vi "FORCE_GUIDE.vi"() -> ()   [LabVIEW 2011]
panel:
  in  "Table":string[][](table)=[["20", "9"], ["30", "6"], ["40", "4.5"]]
  in  "BPM":dbl=20.0 caption="Frequency"
  in  "Boolean":bool
  in  "Filename":path=path "C:/Users/Sinha/Desktop/ULLS/140507-RC.csv"
  in  "Target":bool=TRUE
  in  "GUIDE":bool=TRUE
  in  "AI 1":bool=TRUE
  out "?":bool
  in  "AI 0":bool=TRUE
  in  "Target":dbl=1.25 caption="Offset"
  in  "Sample Rate Hz.":dbl=200.0
  out "Waveform Chart":dbl[][](graph)=[[0.1005629623528339, 0.10453920726000487, 1.25, -0.0], [0.10565121703738356, 0.10453920726000487, 1.25, -0.0], [0.09293058032600965, 0.10453920726000487, 1.25, -0.0], [0.1005629623528339, 0.10453920726000487, 1.25, -0.0], [0.1005629623528339, 0.10453920726000487, 1.25, -0.0], [0.1005629623528339, 0.10453920726000487, 1.25, -0.0], [0.10565121703738356, 0.10453920726000487, 1.25, -0.0], [0.09547470766828448, 0.10453920726000487, 1.25, -0.0], [0.09801883501055919, 0.10453920726000487, 1.25, -0.0], [0.1005629623528339, 0.10453920726000487, 1.25, -0.0], [0.10565121703738356, 0.10453920726000487, 1.25, -0.0], [0.09547470766828436, 0.10453920726000487, 1.25, -0.0], [0.09801883501055919, 0.10453920726000487, 1.25, -0.0], [0.09547470766828448, 0.10453920726000487, 1.25, -0.0], [0.10565121703738356, 0.10453920726000487, 1.25, -0.0], [0.10310708969510873, 0.10453920726000487, 1.25, -0.0], [0.10310708969510873, 0.10453920726000487, 1.25, -0.0], [0.1005629623528339, 0.10453920726000487, 1.25, -0.0], [0.10310708969510873, 0.10453920726000487, 1.25, -0.0], [0.10310708969510873, 0.10453920726000487, 1.25, -0.0]]
  in  "save":bool
  in  "stop (F)":bool caption="stop"
  # "USB"
  # "PCI"
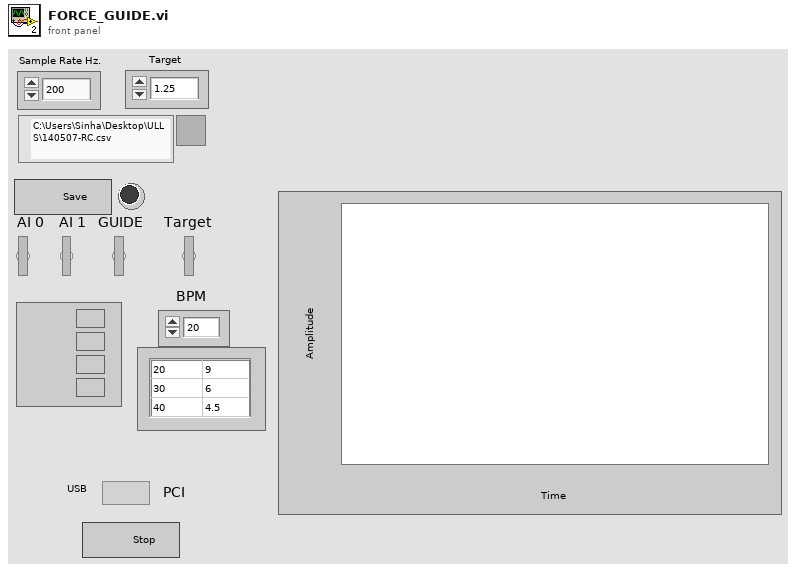
[diagram p1: front panel]
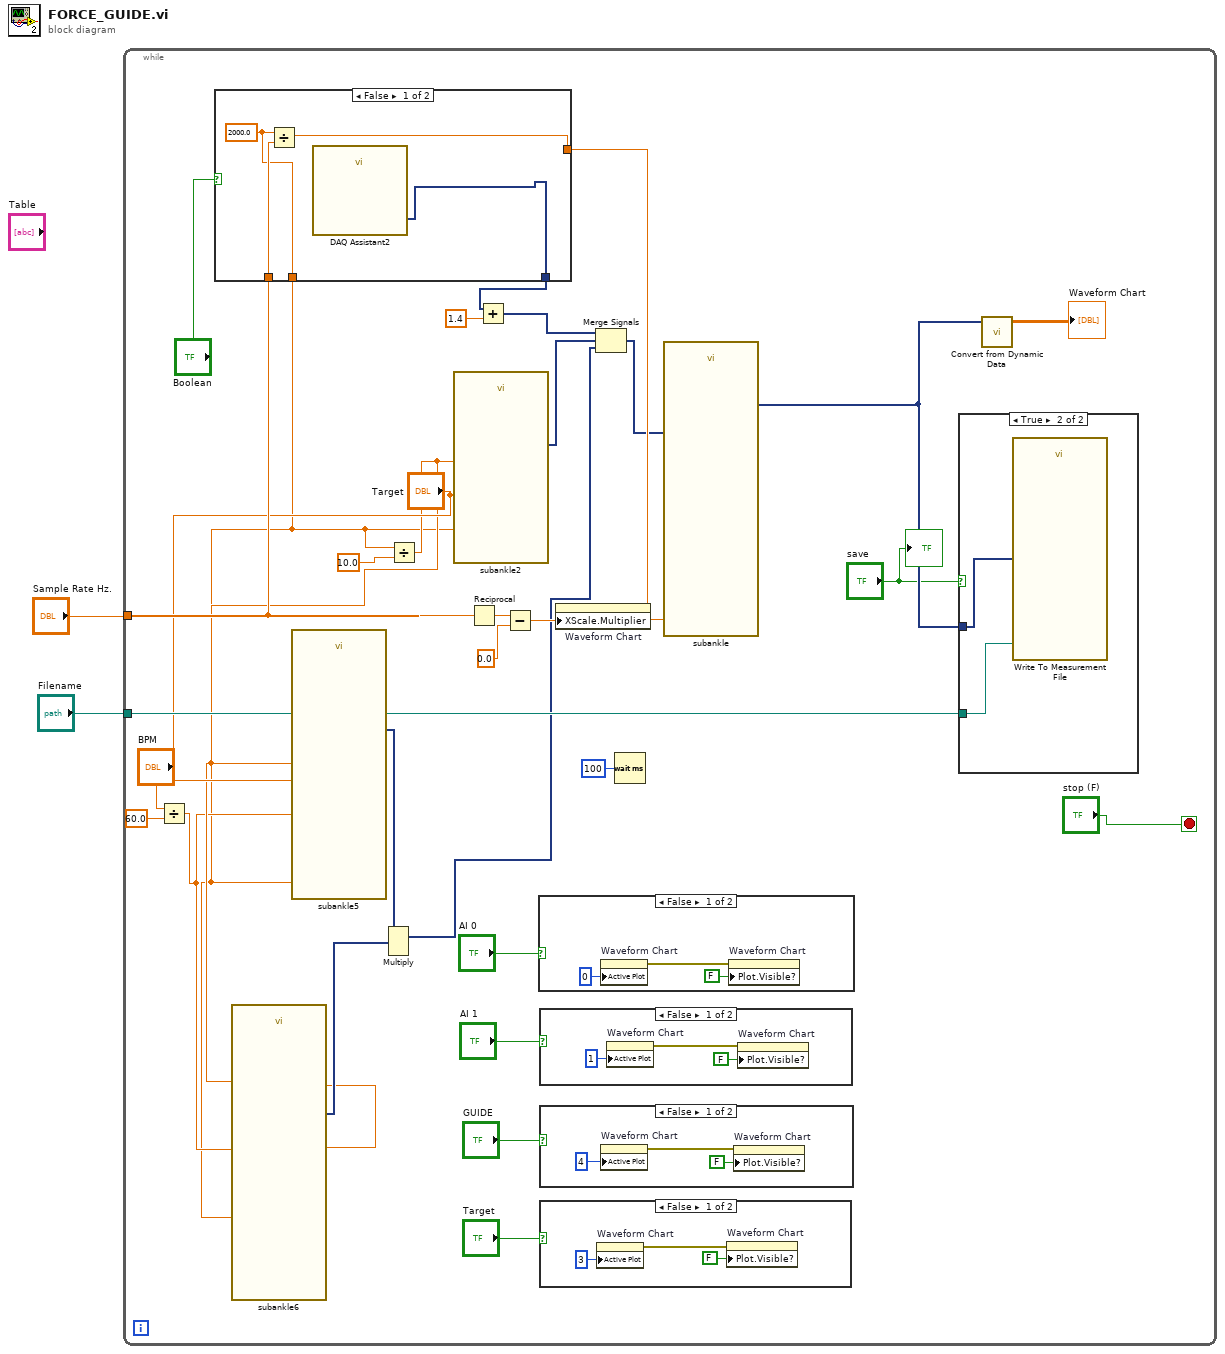
[diagram p0: block diagram]
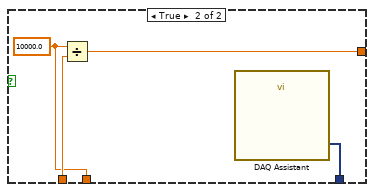
[diagram p2: hidden frame]
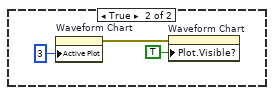
[diagram p3: hidden frame]
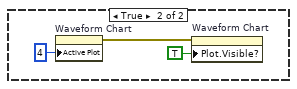
[diagram p4: hidden frame]
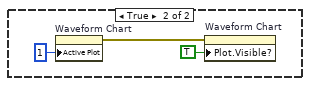
[diagram p5: hidden frame]
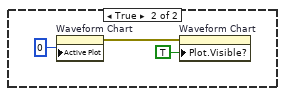
[diagram p6: hidden frame]
diagram:
  n1 = while {
    tunnel: "Sample Rate Hz." -> [w18]
    tunnel: "Filename" -> [w20]
    stop <- "stop (F)" stop-if-true
    n2 = Divide(x="BPM", y=60.0) -> (x/y=w8:dbl)
    n3 = case shown="False" "Boolean" {
      tunnel: [w34 w41] -> w4
      tunnel: w18 -> [w37 w40]
      tunnel: [w36 w39] -> w17
      tunnel: [w35 w38] -> w7
      frame False {
        w35 = 2000.0 ("x")
        n4 = Divide(x=w35, y=w37) -> (x/y=w36:dbl)
        n5 = call "DAQ Assistant2"() -> ("data"=w34:dynamicdata)  [unwired: 16 in, 3 out]
      }
      frame True {
        w38 = 10000.0 ("x")
        n6 = Divide(x=w38, y=w40) -> (x/y=w39:dbl)
        n7 = call "DAQ Assistant"() -> ("data"=w41:dynamicdata)  [unwired: 16 in, 3 out]
      }
    }
    n8 = Divide(x=w7, y=10.0) -> (x/y=w9:dbl)
    n9 = call "subankle6.vi"("Frequency"=w8, "# of Samples"=w9, "Sampling Rate (Hz)"=w7) -> ("Square"=w11:dynamicdata)  [unwired: 11 in, 1 out]
    n10 = call "subankle5.vi"("Frequency"=w8, "Amplitude"="Target", "# of Samples"=w9, "Sampling Rate (Hz)"=w7) -> ("Sine"=w6:dynamicdata)  [unwired: 10 in, 1 out]
    n11 = Multiply(1:w11, 2:w6) -> (0:w15:dynamicdata)  [unwired: 1 in, 1 out]
    n12 = call "subankle2.vi"("Offset"="Target", "# of Samples"=w9, "Sampling Rate (Hz)"=w7) -> ("DC"=w26:dynamicdata)  [unwired: 11 in, 1 out]
    n13 = Reciprocal(x=w18) -> (1/x=w31:dbl)
    n14 = Add(x=w4, y=1.4) -> (x+y=w5:dynamicdata)
    n15 = Subtract(x=w31, y=0.0) -> (x-y=w29:dbl)
    n16 = case shown="False" "AI 0" {
      frame False {
        n17 = property on="Waveform Chart" class="WFChart (strict)"("Active Plot"=u32 0) -> (error out=w61:errorcluster)  [unwired: 2 in, 1 out]
        n18 = property on="Waveform Chart" class="WFChart (strict)"(error in=w61, "Plot.Visible?"=FALSE ("Plot.Visible")) -> ()  [unwired: 1 in, 2 out]
      }
      frame True {
        n19 = property on="Waveform Chart" class="WFChart (strict)"("Active Plot"=u32 0) -> (error out=w64:errorcluster)  [unwired: 2 in, 1 out]
        n20 = property on="Waveform Chart" class="WFChart (strict)"(error in=w64, "Plot.Visible?"=TRUE ("Plot.Visible")) -> ()  [unwired: 1 in, 2 out]
      }
    }
    n21 = case shown="False" "AI 1" {
      frame False {
        n22 = property on="Waveform Chart" class="WFChart (strict)"("Active Plot"=u32 1) -> (error out=w56:errorcluster)  [unwired: 2 in, 1 out]
        n23 = property on="Waveform Chart" class="WFChart (strict)"(error in=w56, "Plot.Visible?"=FALSE ("Plot.Visible")) -> ()  [unwired: 1 in, 2 out]
      }
      frame True {
        n24 = property on="Waveform Chart" class="WFChart (strict)"("Active Plot"=u32 1) -> (error out=w59:errorcluster)  [unwired: 2 in, 1 out]
        n25 = property on="Waveform Chart" class="WFChart (strict)"(error in=w59, "Plot.Visible?"=TRUE ("Plot.Visible")) -> ()  [unwired: 1 in, 2 out]
      }
    }
    n26 = case shown="False" "GUIDE" {
      frame False {
        n27 = property on="Waveform Chart" class="WFChart (strict)"("Active Plot"=u32 4) -> (error out=w50:errorcluster)  [unwired: 2 in, 1 out]
        n28 = property on="Waveform Chart" class="WFChart (strict)"(error in=w50, "Plot.Visible?"=FALSE ("Plot.Visible")) -> ()  [unwired: 1 in, 2 out]
      }
      frame True {
        n29 = property on="Waveform Chart" class="WFChart (strict)"("Active Plot"=u32 4) -> (error out=w52:errorcluster)  [unwired: 2 in, 1 out]
        n30 = property on="Waveform Chart" class="WFChart (strict)"(error in=w52, "Plot.Visible?"=TRUE ("Plot.Visible")) -> ()  [unwired: 1 in, 2 out]
      }
    }
    n31 = case shown="False" "Target" {
      frame False {
        n32 = property on="Waveform Chart" class="WFChart (strict)"("Active Plot"=u32 3) -> (error out=w44:errorcluster)  [unwired: 2 in, 1 out]
        n33 = property on="Waveform Chart" class="WFChart (strict)"(error in=w44, "Plot.Visible?"=FALSE ("Plot.Visible")) -> ()  [unwired: 1 in, 2 out]
      }
      frame True {
        n34 = property on="Waveform Chart" class="WFChart (strict)"("Active Plot"=u32 3) -> (error out=w46:errorcluster)  [unwired: 2 in, 1 out]
        n35 = property on="Waveform Chart" class="WFChart (strict)"(error in=w46, "Plot.Visible?"=TRUE ("Plot.Visible")) -> ()  [unwired: 1 in, 2 out]
      }
    }
    n36 = property on="Waveform Chart" class="WFChart (strict)"("XScale.Multiplier"=w29) -> ()  [unwired: 2 in, 2 out]
    n37 = Merge Signals(w5, w26, w15) -> (w14:dynamicdata)
    n38 = Wait (ms)(milliseconds to wait=u32 100) -> ()  [unwired: 1 out]
    n39 = call "subankle.vi"("Size"=w17, "Signals"=w14) -> ("Median"=w27:dynamicdata)  [unwired: 3 in, 6 out]
    n40 = case shown="True" "save" {
      tunnel: w27 -> [_ w66]
      tunnel: w20 -> [_ w67]
      frame False {
      }
      frame True {
        n41 = call "Write To Measurement File"("Signals"=w66, "Filename"=w67) -> ()  [unwired: 15 in, 3 out]
      }
    }
    n42 = call "Convert from Dynamic Data"("Dynamic Data Type"=w27) -> ("Array"=→"Waveform Chart":dbl[][])  [unwired: 3 in]
    "?" <- "save"
  }
